vi "Test Get Unfiltered Debug Log Not Filtered by Process.vi"(8 "error in (no error)":errorcluster, 11 "Test Case In":refnum<class "Debugger Test.lvclass">) -> (0 "error out":errorcluster, 3 "Test Case Out":refnum<class "Debugger Test.lvclass">)   [LabVIEW 2020, in "Debugger Test.lvclass"]
uses:
  Debugger Test.lvclass
  C:/Program Files (x86)/National Instruments/LabVIEW 2020/vi.lib/Astemes/LUnit/Test Case.lvclass
  source/Debugger/Debugger.lvclass
  C:/Users/anton/Documents/GitHub/triarc-debugger/source/Process/Debug Process.lvclass
  source/Debug Data/Raw Debug Data.ctl
  source/Debug Data/Debug Data.lvclass/Debug Data.ctl
  source/Process/Debug Process.lvclass/Debug Process.ctl
  <vilib>/Astemes/LUnit/Test Case.lvclass/Test Case.ctl
  <vilib>/Astemes/LUnit/LUnit Assertion Result.lvclass/LUnit Assertion Result.ctl
  <vilib>/Astemes/LUnit/LUnit Test Case Result.lvclass/LUnit Test Case Result.ctl
  <vilib>/Astemes/LUnit/LUnit Method Result.lvclass/LUnit Method Result.ctl
  01074fa8-ee8a-411d-bc8b-fc92c4f90959.vi
  <vilib>/AdvancedString/Delimited String to 1D String Array.vi
  source/Process/Public/Lifecycle/Get Lifecycle State.vi
  <vilib>/Astemes/Triarc Framework/Broadcast Event Helpers/Execution timer.vi
  source/Process/Private/SubVIs/Wait for finish.vi
  source/Process/Protected/Messaging/Enqueue Message.vi
  source/Process/Private/SubVIs/Set Lifecycle State.vi
  <vilib>/Astemes/LUnit/Palette/Pass.vi
  <vilib>/Astemes/LUnit/Palette/Fail.vi
  <vilib>/Astemes/LUnit/Compare Variants.vi
  <vilib>/Astemes/LUnit/Describe Comparison.vi
  <vilib>/Astemes/LUnit/Set Assertion Type.vi
  <vilib>/Utility/error.llb/Clear Errors.vi
  <vilib>/Astemes/LUnit/Add test result.vi
  <vilib>/Astemes/LUnit/LUnit Write Passed.vi
  <vilib>/Astemes/LUnit/LUnit Write Message.vi
  <vilib>/Astemes/LUnit/LUnit Write Description.vi
  <vilib>/Astemes/LUnit/Variant to string.vi
  <vilib>/Astemes/LUnit/LUnit Write Assertion Type.vi
  <vilib>/Astemes/LUnit/LUnit Record Assertion Result.vi
  <vilib>/Astemes/LUnit/LUnit Aggregate Assertion Results.vi
  <vilib>/Astemes/LUnit/Assertion Result/LUnit Read Status.vi
  <vilib>/Astemes/LUnit/LUnit Read Message.vi
  <vilib>/Astemes/LUnit/LUnit Read Description.vi
  <vilib>/Astemes/LUnit/Method Result/LUnit Merge Status.vi
  <vilib>/Astemes/LUnit/LUnit Concatenate result strings.vi
  <vilib>/Utility/error.llb/Error Cluster From Error Code.vi
  <vilib>/Astemes/Triarc Framework/Broadcast Event Helpers/Dequeue Broadcast Message.vi
  <vilib>/Utility/Data Type/Get Type Information.vi
  <vilib>/Utility/LVClass/Get LV Class Name.vi
  source/Debug Data/Debug Data.lvclass
  <vilib>/Astemes/LUnit/LUnit Assertion Result.lvclass
  source/Process/Debug Process.lvclass
  <vilib>/Astemes/Triarc Framework/Broadcast Event Helpers/Broadcast Event Helpers.lvlib
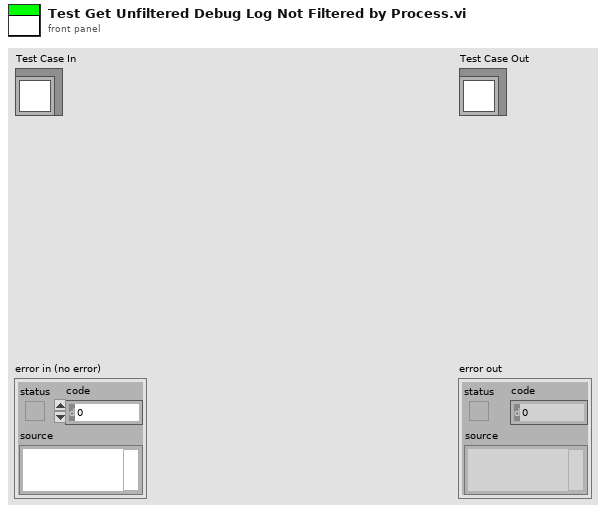
[diagram p1: front panel]
types:
  T1 = typedef "Debug Data.lvclass/Raw Debug Data.ctl" = cluster{"Action":string, "Call Chain":string, "Process":string, "Message":string, "Message Data":variant, "Time":dbl}
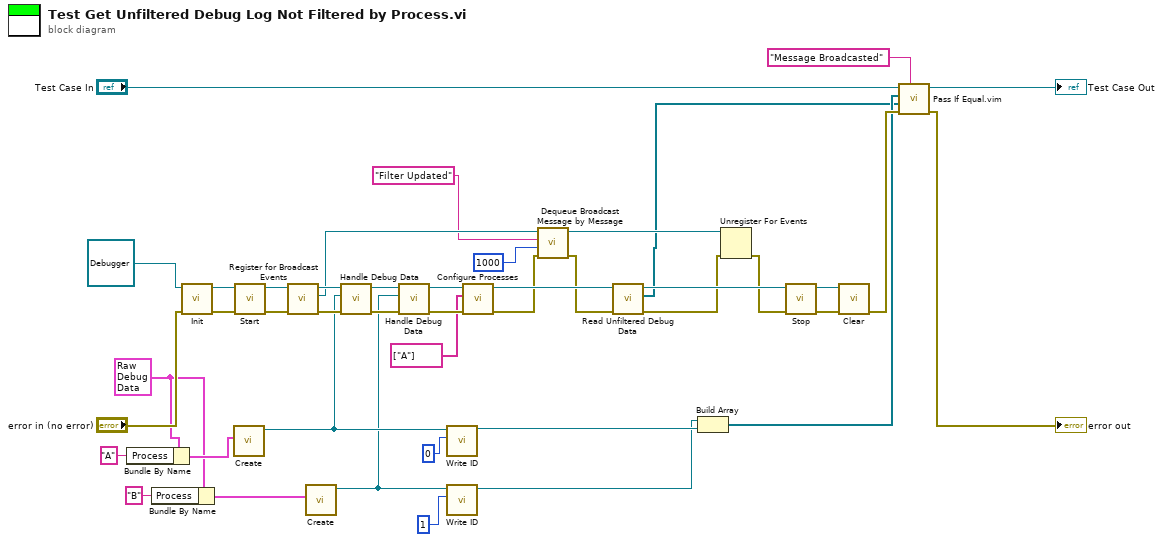
[diagram p0: block diagram]
diagram:
  w18 = T1 {"Action"="", "Call Chain"="", "Process"="", "Message"="", "Message Data"=variant, "Time"=0.0} ("Debug Data Cluster")
  n1 = Bundle By Name(cluster=w18, "Process"="A") -> (w25:T1)
  n2 = Bundle By Name(cluster=w18, "Process"="B") -> (w19:T1)
  n3 = call-dynamic "Init.vi"("error in (no error)"="error in (no error)", "Process In"=refnum<class "Debugger.lvclass"> refnum ("Debug Data Event In 2")) -> ("error out"=w39:errorcluster, "Process Out"=w40:refnum<class "Debugger.lvclass">)  [unwired: 8 in]
  n4 = call "Create.vi"("Debug Data Cluster"=w25) -> ("Debug Data out"=w8:refnum<class "Debug Data.lvclass">)  [unwired: 9 in, 1 out]
  n5 = call "Start.vi"("error in (no error)"=w39, "Process In"=w40) -> ("error out"=w37:errorcluster, "Process Out"=w38:refnum<class "Debugger.lvclass">)  [unwired: 7 in, 1 out]
  n6 = call "Register for Broadcast Events.vi"("error in (no error)"=w37, "Process In"=w38) -> ("error out"=w36:errorcluster, "Event Registration Refnum Out"=w26:refnum<event-registration>, "Process Out"=w32:refnum<class "Debugger.lvclass">)  [unwired: 7 in]
  n7 = call "Create.vi"("Debug Data Cluster"=w19) -> ("Debug Data out"=w7:refnum<class "Debug Data.lvclass">)  [unwired: 9 in, 1 out]
  n8 = call-dynamic "Handle Debug Data.vi"("error in (no error)"=w36, "Debug Data.lvclass"=w8, "Debug Data Event In"=w32) -> ("error out"=w22:errorcluster, "Debug Data Event Out"=w23:refnum<class "Debugger.lvclass">)  [unwired: 7 in]
  n9 = call-dynamic "Handle Debug Data.vi"("error in (no error)"=w22, "Debug Data.lvclass"=w7, "Debug Data Event In"=w23) -> ("error out"=w21:errorcluster, "Debug Data Event Out"=w17:refnum<class "Debugger.lvclass">)  [unwired: 7 in]
  n10 = call "Write ID.vi"("ID"=u32 0, "Debug Data in"=w8) -> ("Debug Data out"=w12:refnum<class "Debug Data.lvclass">)  [unwired: 8 in, 1 out]
  n11 = call "Write ID.vi"("ID"=u32 1, "Debug Data in"=w7) -> ("Debug Data out"=w11:refnum<class "Debug Data.lvclass">)  [unwired: 8 in, 1 out]
  n12 = call "Configure Processes.vi"("error in (no error)"=w21, "Processes"=string[] ["A"], "Debugger In"=w17) -> ("error out"=w2:errorcluster, "Debugger Out"=w16:refnum<class "Debugger.lvclass">)  [unwired: 7 in]
  n13 = call <vilib>:"Dequeue Broadcast Message by Message.vi"("error in (no error)"=w2, "Timeout (-1)"=1000, "Message"="Filter Updated", "Event Registration Refnum"=w26) -> ("error out"=w1:errorcluster, "Event Registration Refnum Out"=w6:refnum<event-registration>)  [unwired: 3 in, 3 out]
  n14 = call "Read Unfiltered Debug Data.vi"("error in (no error)"=w1, "Debugger In"=w16) -> ("error out"=w14:errorcluster, "Data Log"=w3:refnum<class "Debug Data.lvclass">[], "Debugger Out"=w35:refnum<class "Debugger.lvclass">)  [unwired: 7 in]
  n15 = Build Array(w11, w12) -> (w27:refnum<class "Debug Data.lvclass">[])
  n16 = Unregister For Events(event registration refnum=w6, error in=w14) -> (error out=w13:errorcluster)
  n17 = call "Stop.vi"("error in (no error)"=w13, "Process In"=w35) -> ("error out"=w33:errorcluster, "Process Out"=w34:refnum<class "Debugger.lvclass">)  [unwired: 7 in, 1 out]
  n18 = call-dynamic "Clear.vi"("error in (no error)"=w33, "Process In"=w34) -> ("error out"=w29:errorcluster)  [unwired: 9 in]
  n19 = call "Pass If Equal.vim"("Description"="Message Broadcasted", "error in (no error)"=w29, "Actual"=w3, "Expected"=w27, "LUnit Test Case In"="Test Case In") -> ("error out"=→"error out":errorcluster, "LUnit Test Case Out"=→"Test Case Out":refnum<class "Debugger Test.lvclass">)  [unwired: 5 in]
